vi "Mutate_v1_to_v2.vi"(11 "SerializableData_v1":T2) -> (0 "error out":errorcluster, 3 "SerializableData":T1)   [LabVIEW 2019, in "Bill Murray.lvclass"]
uses:
  Bill Murray.lvclass
  SerializableData_v1.ctl
  Golf Club.lvclass
  SerializableData.ctl
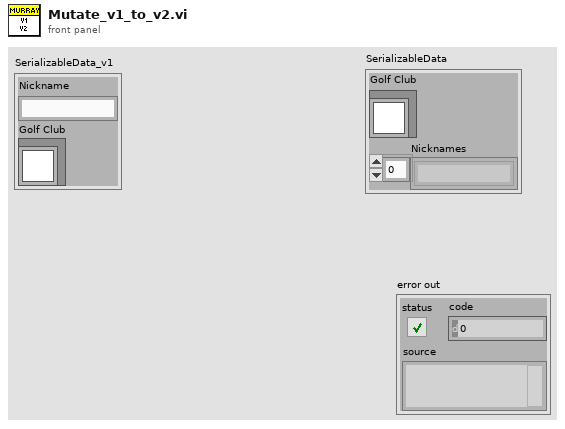
[diagram p1: front panel]
types:
  T1 = typedef "Bill Murray.lvclass/SerializableData.ctl" = cluster{"Golf Club":refnum<class "Golf Club.lvclass">, "Nicknames":string[]}
  T2 = typedef "Bill Murray.lvclass/SerializableData_v1.ctl" = cluster{"Nickname":string, "Golf Club":refnum<class "Golf Club.lvclass">}
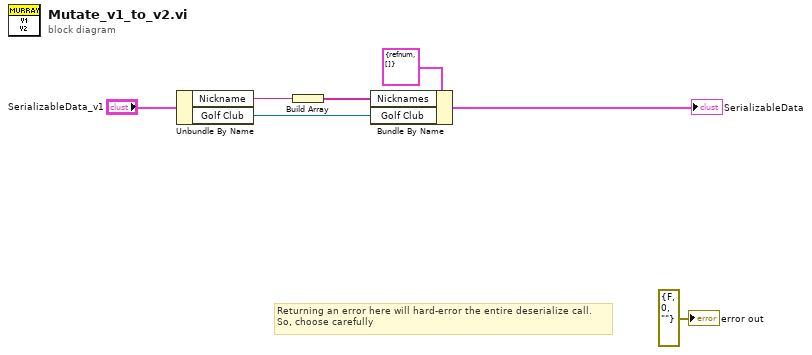
[diagram p0: block diagram]
diagram:
  # "Returning an error here will hard-error the entire deserialize call.\nSo, choose carefully"
  n1 = Unbundle By Name("SerializableData_v1") -> ("Nickname"=w4:string, "Golf Club"=w2:refnum<class "Golf Club.lvclass">)
  n2 = Build Array(w4) -> (w3:string[])
  n3 = Bundle By Name(cluster=T1 {"Golf Club"=refnum, "Nicknames"=[]} ("SerializableData"), "Nicknames"=w3, "Golf Club"=w2) -> (→"SerializableData":T1)
  "error out" <- errorcluster {"status"=FALSE, "code"=0, "source"=""} ("error out")
